vi "Read queue.vi"(8 "error in (no error)":errorcluster, 11 "mqtt in":refnum<class "mqtt.lvclass">) -> (0 "error out":errorcluster, 2 "queue":refnum<queue>, 3 "mqtt out":refnum<class "mqtt.lvclass">)   [LabVIEW 2018, in "labview-mqtt.lvlib" / "mqtt.lvclass"]
uses:
  mqtt.lvclass
  mqtt.lvclass/mqtt.ctl
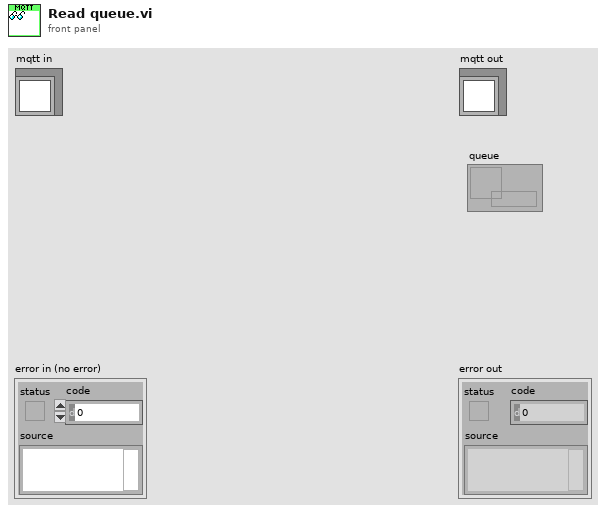
[diagram p1: front panel]
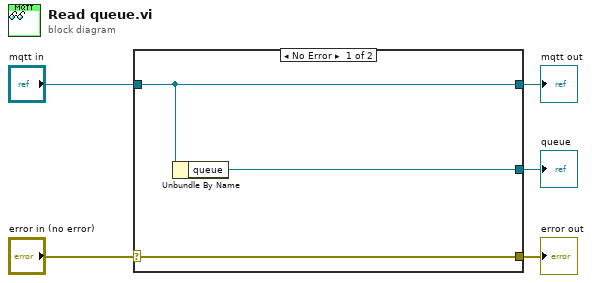
[diagram p0: block diagram]
diagram:
  n1 = case shown="No Error" "error in (no error)" {
    selector: "error in (no error)" -> [w8 w9]
    tunnel: [w8 w9] -> w4
    tunnel: [w7 w10] -> w2
    tunnel: "mqtt in" -> [w7 w10]
    tunnel: [w6 _] -> w1
    frame No Error {
      n2 = Unbundle By Name(w7) -> ("queue"=w6:refnum<queue>)
    }
    frame Error {
    }
  }
  "error out" <- w4
  "mqtt out" <- w2
  "queue" <- w1
